vi "Get all results as 2D strings array.vi"(8 "error in (no error)":errorcluster, 11 "PQ Result in":refnum<class "PQ Result.lvclass">) -> (0 "error out":errorcluster, 2 "Strings":string[][](array[string]), 3 "PQ Result out":refnum<class "PQ Result.lvclass">)   [LabVIEW 2016, in "PQ Result.lvclass"]
uses:
  PQ Result.lvclass
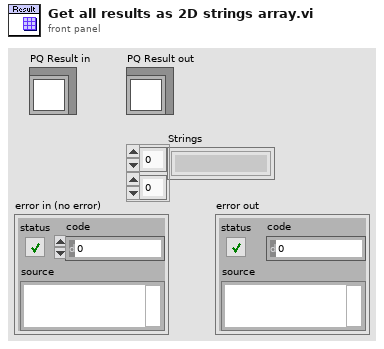
[diagram p1: front panel]
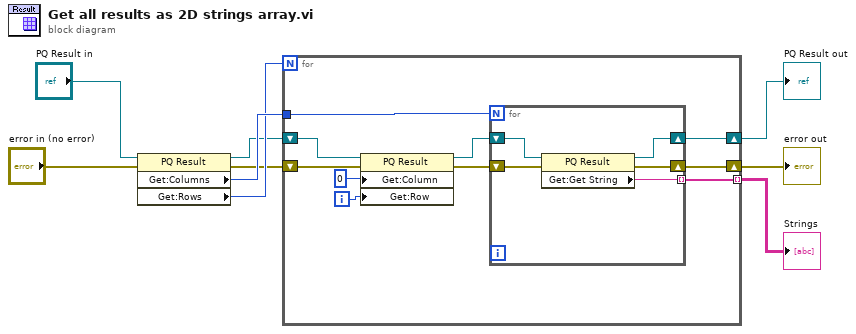
[diagram p0: block diagram]
diagram:
  n1 = property class="PQ Result"(reference="PQ Result in", error in="error in (no error)") -> (reference out=w6:refnum<class "PQ Result.lvclass">, error out=w2:errorcluster, "Get:Columns"=w9:i32, "Get:Rows"=w7:i32)
  n2 = for {
    N: w7 -> [_]
    shift-right: [w15] -> w8
    shift-left: w6 -> [w19]
    tunnel: [w14] -> w5 mode=indexing
    tunnel: w9 -> [w13]
    shift-right: [w10] -> w1
    shift-left: w2 -> [w12]
    i -> [w18]
    n3 = property class="PQ Result"(reference=w19, error in=w12, "Get:Column"=0 ("Next Column"), "Get:Row"=w18) -> (reference out=w16:refnum<class "PQ Result.lvclass">, error out=w11:errorcluster)
    n4 = for {
      N: w13 -> [_]
      shift-right: [w23] -> w15
      shift-left: w16 -> [w24]
      tunnel: [w22] -> w14 mode=indexing
      shift-right: [w20] -> w10
      shift-left: w11 -> [w21]
      n5 = property class="PQ Result"(reference=w24, error in=w21) -> (reference out=w23:refnum<class "PQ Result.lvclass">, error out=w20:errorcluster, "Get:Get String"=w22:string)
    }
  }
  "PQ Result out" <- w8
  "Strings" <- w5
  "error out" <- w1
